vi "ClockListener.vi"   [LabVIEW 2009]
uses:
  <vilib>/lvdsc/NI_DSC.lvlib
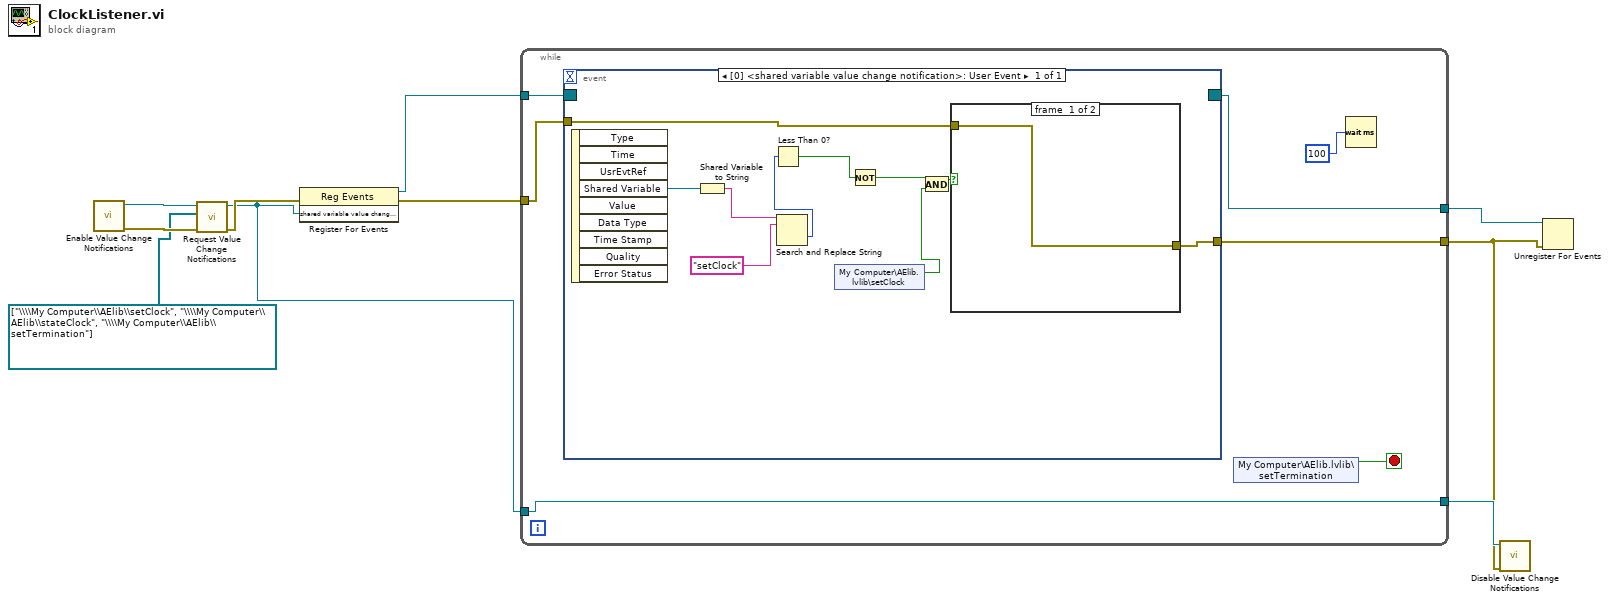
[diagram p0: block diagram]
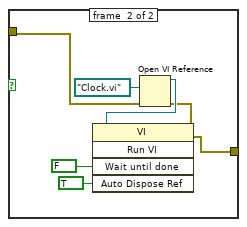
[diagram p2: hidden frame]
diagram:
  n1 = call <vilib>:"Enable Value Change Notifications.vi"() -> ("error out"=w10:errorcluster, "shared variable value change notification"=w9:refnum<user-event>)  [unwired: 10 in]
  n2 = call <vilib>:"Request Value Change Notifications.vi"("error in (no error)"=w10, "shared variables"=refnum<k21>[] ["\\\\My Computer\\AElib\\setClock", "\\\\My Computer\\AElib\\stateClock", "\\\\My Computer\\AElib\\setTermination"], "notification refnum"=w9) -> ("error out"=w7:errorcluster, "shared variable value change notification"=w4:refnum<user-event>)  [unwired: 6 in, 1 out]
  n3 = register-events(error in=w7, w4) -> (reference out=w6:refnum<event-registration>, error out=w3:errorcluster)  [unwired: 1 in]
  n4 = while {
    tunnel: w6 -> [w17]
    tunnel: [w16] -> w5
    tunnel: w4 -> [w15]
    tunnel: w3 -> [w13]
    tunnel: [w15] -> w2
    tunnel: [w12] -> w1
    stop <- w11 stop-if-true
    n5 = event shown="[0] <shared variable value change notification>: User Event" {
      selector: w17 -> [_]
      dyn-events: [_] -> w16
      timeout: _ -> [_]
      tunnel: w13 -> [w23]
      tunnel: [w22] -> w12
      event [0] <shared variable value change notification>: User Event {
        n6 = event-data() -> ("Shared Variable"=w27:refnum<k21>)  [unwired: 1 in, 8 out]
        n7 = Shared Variable to String(1:w27) -> (0:w26:string)
        n8 = Search and Replace String(input string=w26, search string="setClock") -> (offset past replacement=w24:i32)  [unwired: 6 in, 3 out]
        n9 = Less Than 0?(x=w24) -> (x < 0?=w20:bool)
        n10 = shared-variable "My Computer\\AElib.lvlib\\setClock"() -> (w19:bool)  [unwired: 1 in, 1 out]
        n11 = Not(x=w20) -> (.not. x?=w18:bool)
        n12 = And(x=w18, y=w19) -> (x .and. y?=w21:bool)
        n13 = case shown="False" w21 {
          tunnel: w23 -> [w28 w30]
          tunnel: [w28 w29] -> w22
          frame #0 {
          }
          frame #1 {
            n14 = Open VI Reference(vi path=path "Clock.vi", error in (no error)=w30) -> (vi reference=w34:refnum<vi>, error out=w33:errorcluster)  [unwired: 4 in]
            n15 = invoke class="VI" method="Run VI"(reference=w34, error in=w33, "Wait until done"=FALSE, "Auto Dispose Ref"=TRUE ("Auto Dispose Reference")) -> (error out=w29:errorcluster)  [unwired: 1 in, 4 out]
          }
        }
      }
    }
    n16 = shared-variable "My Computer\\AElib.lvlib\\setTermination"() -> (w11:bool)  [unwired: 1 in, 1 out]
    n17 = Wait (ms)(milliseconds to wait=u32 100) -> ()  [unwired: 1 out]
  }
  n18 = call <vilib>:"Disable Value Change Notifications.vi"("error in (no error)"=w1, "notification refnum"=w2) -> ()  [unwired: 9 in, 1 out]
  n19 = Unregister For Events(event registration refnum=w5, error in=w1) -> ()  [unwired: 1 out]
